vi "InitiateGeneration.vi"(8 "error in (no error)":errorcluster, 11 "NiPxi6733 in":refnum<class "NiPxi6733.lvclass">) -> (0 "error out":errorcluster, 3 "NiPxi6733 out":refnum<class "NiPxi6733.lvclass">)   [LabVIEW 2014, in "FgenPlugins.lvlib" / "NiPxi6733.lvclass"]
uses:
  NiPxi6733.lvclass
  FgenPluginBaseClass/FgenPluginsBase.lvclass/FgenPluginsBase.ctl
  MemberClasses/FunctionBaseClass/FunctionBase.lvclass/FunctionBase.ctl
  FgenPluginBaseClass/Accessors/Read Channels.vi
  FgenPluginBaseClass/Accessors/Read FunctionClass.vi
  MemberClasses/FunctionBaseClass/Accessors/Read Waveforms.vi
  <vilib>/DAQmx/write.llb/DAQmx Write (Analog 1D Wfm NChan NSamp).vi
  MemberClasses/FunctionBaseClass/FunctionBase.lvclass
panel:
  out "NumSamples":u32
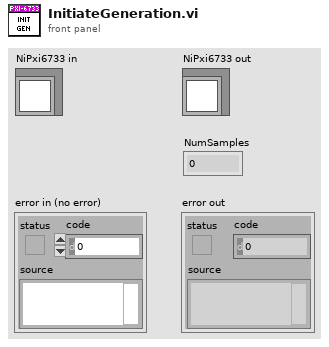
[diagram p1: front panel]
types:
  T1 = typedef "FgenPlugins.lvlib/Channel.ctl" = cluster{"Name":string, "Enabled":bool, "Operation":enum16{"Continuous", "Burst"}, "Impedance (50)":dbl, "Handle":string, "Connected":bool, "Mode (Function)":enum16{"Function", "Arbitrary", "Sequence"}}
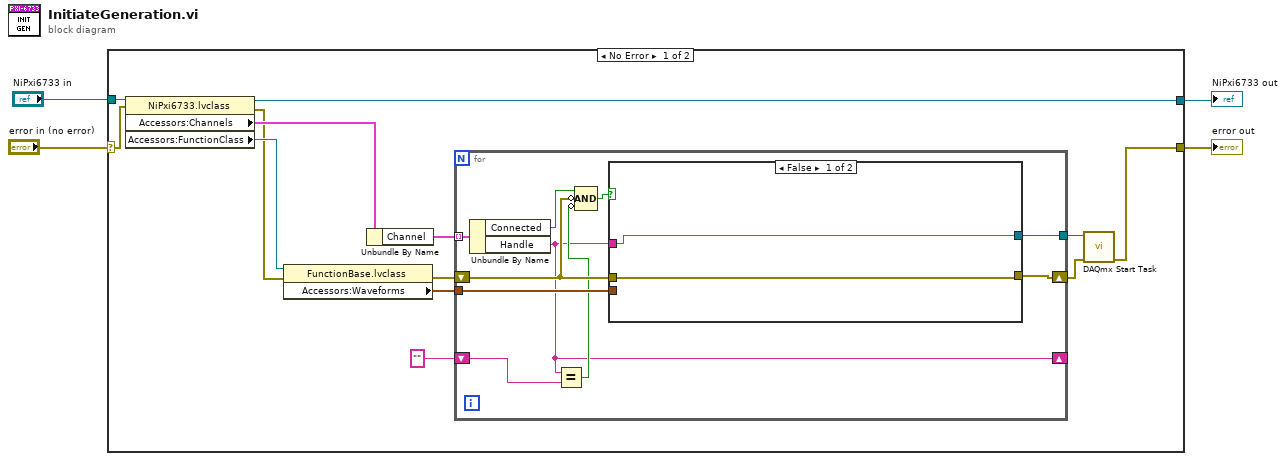
[diagram p0: block diagram]
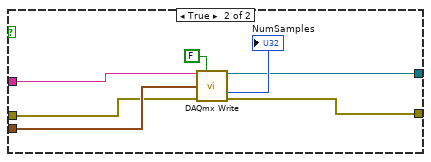
[diagram p2: hidden frame]
diagram:
  n1 = case shown="No Error" "error in (no error)" {
    selector: "error in (no error)" -> [w15 w37]
    tunnel: "NiPxi6733 in" -> [w17 w38]
    tunnel: [w9 w38] -> w2
    tunnel: [w5 w37] -> w1
    frame No Error {
      n2 = property class="NiPxi6733.lvclass"(reference=w17, error in=w15) -> (reference out=w9:refnum<class "NiPxi6733.lvclass">, error out=w11:errorcluster, "Accessors:Channels"=w16:cluster{"Count":u16, "Channel":T1[]}, "Accessors:FunctionClass"=w13:refnum<class "FunctionBase.lvclass">)
      n3 = property class="FunctionBase.lvclass"(reference=w13, error in=w11) -> (error out=w10:errorcluster, "Accessors:Waveforms"=w12:waveform(dbl)[])  [unwired: 1 out]
      n4 = Unbundle By Name(w16) -> ("Channel"=w14:T1[])
      n5 = for {
        tunnel: w14 -> [w27] mode=indexing
        tunnel: w12 -> [w26]
        shift-right: [w22] -> w6
        shift-left: w10 -> [w24]
        shift-right: [w19] -> _
        shift-left: "" -> [w21]
        tunnel: [w18] -> w7
        n6 = Unbundle By Name(w27) -> ("Connected"=w25:bool, "Handle"=w19:string)
        n7 = Equal?(x=w19, y=w21) -> (x = y?=w20:bool)
        n8 = Compound Arithmetic op=AND(w25, invert w24, invert w20) -> (w23:bool)
        n9 = case shown="False" w23 {
          tunnel: w26 -> [_ w35]
          tunnel: w24 -> [w29 w34]
          tunnel: [w29 w32] -> w22
          tunnel: w19 -> [w28 w31]
          tunnel: [w28 w30] -> w18
          frame False {
          }
          frame True {
            n10 = call-poly <vilib>:"DAQmx Write.vi"("task/channels in"=w31, "auto start"=FALSE, "data"=w35, "error in"=w34) -> ("task out"=w30:refnum<k21>, "number of samples written per channel"=→"NumSamples":u32, "error out"=w32:errorcluster)  [unwired: 9 in]
          }
        }
      }
      n11 = call <vilib>:"DAQmx Start Task.vi"("task/channels in"=w7, "error in"=w6) -> ("error out"=w5:errorcluster)  [unwired: 12 in, 1 out]
    }
    frame Error {
    }
  }
  "error out" <- w1
  "NiPxi6733 out" <- w2
